vi "Hembras.vi"() -> ()   [LabVIEW 2013]
doc: "This example performs a serial port write and a serial port read. The parameters set for the serial port must match the parameters of the connected instrument or device. The VISA Configure Serial Port VI sets the configuration parameters. The front panel displays the controls used to configure the basic parameters, such as baud rate, data bits, and parity. The VI passes the VISA resource name to other VIs that perform operations on that VISA resource. The VISA Write function sends a command to the serial device and the VISA Read function returns data based on the command. The VISA Close function then closes the reference to the serial device. It is important to close the reference; otherwise, further communication through that port might not be possible."
uses:
  <vilib>/Platform/TimedLoop/XDataNode/timing_clust.ctl
  <vilib>/Platform/TimedLoop/XDataNode/nitl_modes.ctl
  <vilib>/Platform/TimedLoop/XDataNode/wakeup.ctl
  <vilib>/Instr/_visa.llb/VISA Configure Serial Port (Instr).vi
  <vilib>/Utility/file.llb/Read From Spreadsheet File (I64).vi
  <vilib>/platform/TimedLoop/XDataNode/XDataNode.xnode
  <vilib>/Platform/TimedLoop/XDataNode/XDNodeRunTimeDep.lvlib
panel:
  in  "Puerto":refnum<visa-resource-name>
  out "Entradas":u8[][](array[numeric])
  in  "Abrir arnés":bool
  out "Test":bool
  out "Bien?":bool[][](array[boolean])
  out "Entradas Testeadas":u8[][](array[numeric])
  out "Salidas":u8[](array[numeric])
  out "OK?":bool
  in  "stop":bool
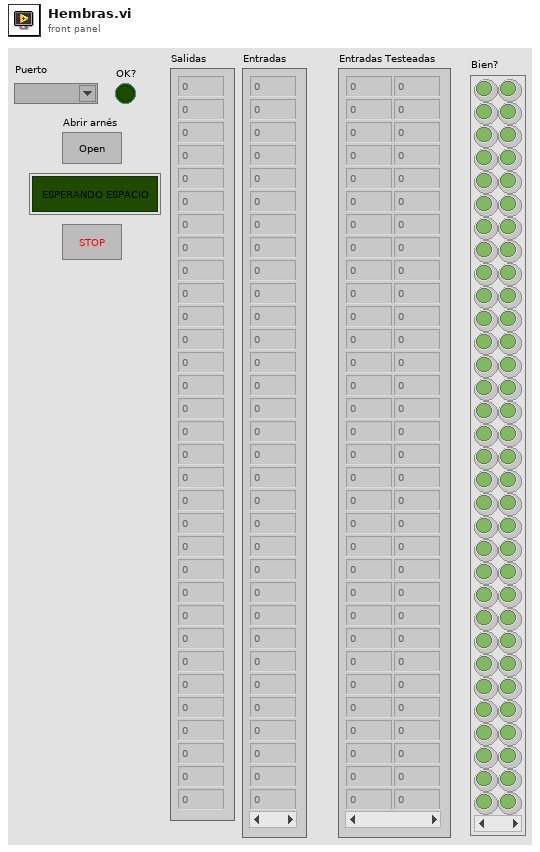
[diagram p1: front panel]
types:
  T1 = typedef "XDNodeRunTimeDep.lvlib/timing_clust.ctl" = cluster{"Expected End [f-1]":u64, "Actual End [f-1]":u64, "Finished Late? [f-1]":bool, "Expected End [i-1]":u64, "Actual End [i-1]":u64, "Finished Late? [i-1]":bool, "Expected Start [i]":u64, "Actual Start [i]":u64, "Expected Start [f]":u64, "Actual Start [f]":u64, "Source Name":string, "Structure Name":string, "Period":i64, "Deadline":i64, "Offset":i64, "Start":i64, "Priority":i32, "Timeout":i32, "Mode":T2, "Wakeup Reason":T3, "Error":errorcluster, "Source Type":string, "Secondary Source Type":string, "Global End Time":u64, "Global Start Time":u64, "Frame Duration":u64, "Iteration Duration":u64, "Assigned CPU":i32, "I/O Scan Engine Mode":u32}
  T2 = typedef "XDNodeRunTimeDep.lvlib/nitl_modes.ctl" = enum32{"No Change", "Process missed periods, maintain original phase", "Discard missed periods, maintain original phase", "Process missed periods, ignore original phase", "Discard missed periods, ignore original phase"}
  T3 = typedef "XDNodeRunTimeDep.lvlib/wakeup.ctl" = enum32{"Normal", "Aborted", "Asynchronous wakeup", "Timing source error", "Timed loop error", "Timeout"}
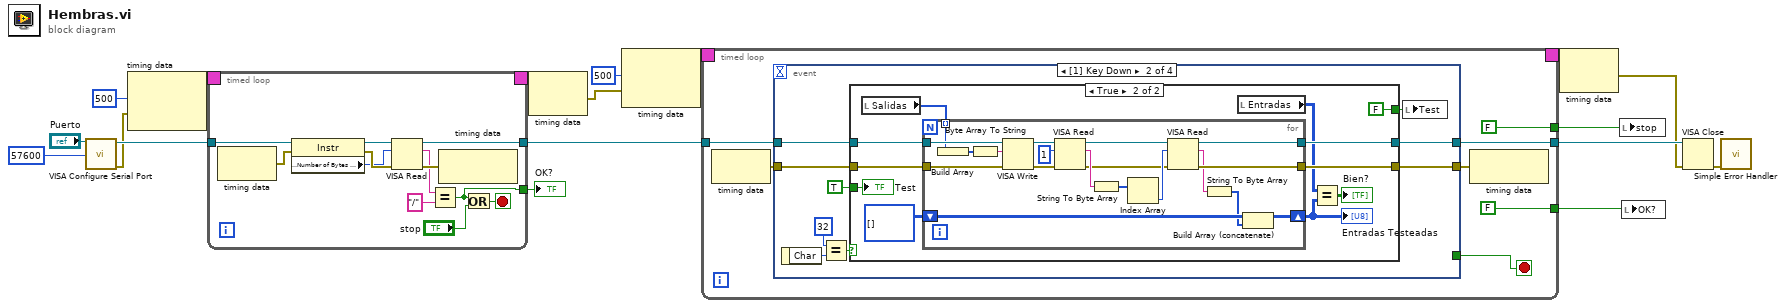
[diagram p0: block diagram]
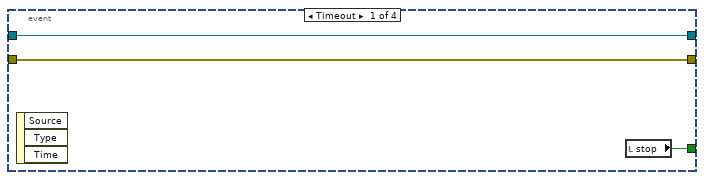
[diagram p2: hidden frame]
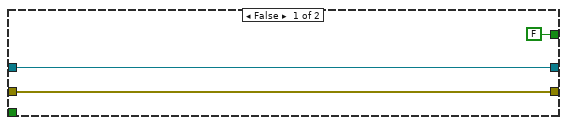
[diagram p3: hidden frame]
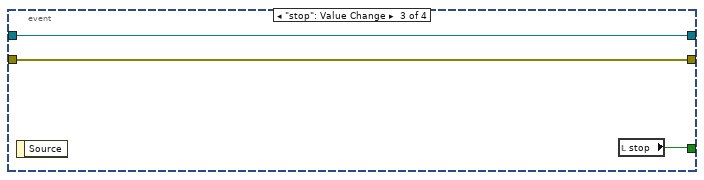
[diagram p4: hidden frame]
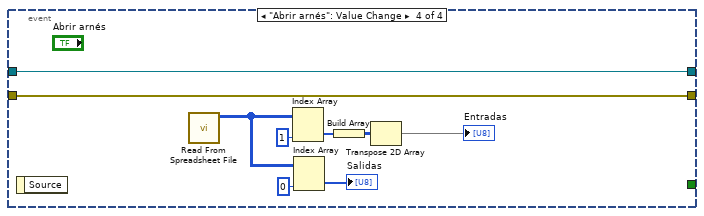
[diagram p5: hidden frame]
diagram:
  n1 = call-poly "VISA Configure Serial Port"("VISA resource name"="Puerto", "baud rate (9600)"=u32 57600) -> ("VISA resource name out"=w18:refnum<visa-resource-name>, "error out"=w15:errorcluster)  [unwired: 7 in, 5 out]
  n2 = node-c288(i64 500 ("Period"), w15) -> (w17:T1)
  n3 = timed-loop {
    timing: w17 -> [_]
    timing-out: [_] -> w16
    tunnel: [w30] -> w5
    tunnel: w18 -> [w29]
    tunnel: [w19] -> w8
    stop <- w20 stop-if-true
    n4 = node-c288() -> (w25:errorcluster)  [unwired: 1 in]
    n5 = property class="Instr"(reference=w29, error in=w25) -> (reference out=w28:refnum<visa-resource-name>, error out=w27:errorcluster, "Serial Settings:Number of Bytes at Serial Port"=w26:u32)
    n6 = VISA Read(VISA resource name=w28, byte count=w26, error in (no error)=w27) -> (VISA resource name out=w30:refnum<visa-resource-name>, read buffer=w23:string, error out=w24:errorcluster)  [unwired: 1 out]
    n7 = Equal?(x=w23, y="/") -> (x = y?=w19:bool)
    n8 = node-c288(w24) -> ()  [unwired: 1 out]
    n9 = Or(x=w19, y="stop") -> (x .or. y?=w20:bool)
  }
  "OK?" <- w8
  n10 = node-c288(w16) -> (w4:errorcluster)
  n11 = node-c288(i64 500 ("Period"), w4) -> (w11:T1)
  n12 = timed-loop {
    timing: w11 -> [_]
    timing-out: [_] -> w10
    tunnel: w5 -> [w42]
    tunnel: [FALSE ("stop")] -> w12
    tunnel: [w40] -> w3
    tunnel: [FALSE ("OK?")] -> w7
    stop <- w36 stop-if-true
    n13 = node-c288() -> (w39:errorcluster)  [unwired: 1 in]
    n14 = event shown="[1] Key Down" {
      selector: _ -> [_ _ _ _]
      dyn-events: _ -> [_ _ _ _]
      timeout: _ -> [_ _ _ _]
      tunnel: w42 -> [w44 w54 w89 w92]
      tunnel: [w44 w53 w89 w92] -> w40
      tunnel: w39 -> [w43 w52 w88 w91]
      tunnel: [w43 w51 w88 w91] -> w38
      tunnel: [w45 _ w90 _] -> w36
      event Timeout {
        n15 = event-data() -> ()  [unwired: 1 in, 3 out]
        n16 = local read "stop"() -> (w45:bool)
      }
      event Key Down {
        n17 = event-data() -> ("Char"=w49:i16)  [unwired: 1 in]
        n18 = Equal?(x=i16 32, y=w49) -> (x = y?=w50:bool)
        n19 = case shown="True" w50 {
          tunnel: w54 -> [w57 w68]
          tunnel: [w57 w65] -> w53
          tunnel: w52 -> [w56 w67]
          tunnel: [w56 w66] -> w51
          tunnel: TRUE -> [_ w61]
          tunnel: [FALSE FALSE] -> w46
          frame False {
          }
          frame True {
            n20 = local read "Salidas"() -> (w58:u8[])
            n21 = for {
              tunnel: w68 -> [w87]
              tunnel: w67 -> [w85]
              tunnel: [w77] -> w66
              tunnel: [w76] -> w65
              shift-right: [w74] -> w62
              shift-left: i32[][] [] -> [w73]
              tunnel: w58 -> [w69] mode=indexing
              n22 = Build Array(w69) -> (w71:u8[])
              n23 = Byte Array To String ("Byte Array \nTo String")(unsigned byte array=w71) -> (string=w70:string)
              n24 = VISA Write(VISA resource name=w87, write buffer=w70, error in (no error)=w85) -> (VISA resource name out=w84:refnum<visa-resource-name>, error out=w83:errorcluster)  [unwired: 1 out]
              n25 = VISA Read(VISA resource name=w84, byte count=u32 1, error in (no error)=w83) -> (VISA resource name out=w78:refnum<visa-resource-name>, read buffer=w86:string, error out=w79:errorcluster)  [unwired: 1 out]
              n26 = String To Byte Array(string=w86) -> (unsigned byte array=w81:u8[])
              n27 = Index Array(array=w81) -> (element=w80:u8)  [unwired: 1 in]
              n28 = VISA Read(VISA resource name=w78, byte count=w80, error in (no error)=w79) -> (VISA resource name out=w76:refnum<visa-resource-name>, read buffer=w75:string, error out=w77:errorcluster)  [unwired: 1 out]
              n29 = String To Byte Array(string=w75) -> (unsigned byte array=w72:u8[])
              n30 = Build Array (concatenate)(w73, w72) -> (w74:i32[][])
            }
            "Entradas Testeadas" <- w62
            n31 = local read "Entradas"() -> (w59:u8[][])
            n32 = Equal?(x=w59, y=w62) -> (x = y?=→"Bien?":bool[][])
            "Test" <- w61
          }
        }
        n33 = local write "Test"(w46) -> ()
      }
      event "stop": Value Change {
        n34 = event-data() -> ()  [unwired: 1 in, 1 out]
        n35 = local read "stop"() -> (w90:bool)
      }
      event "Abrir arnés": Value Change {
        n36 = event-data() -> ()  [unwired: 1 in, 1 out]
        n37 = call-poly <vilib>:"Read From Spreadsheet File.vi"() -> ("all rows"=w95:i64[][])  [unwired: 7 in, 4 out]
        n38 = Index Array(array=w95, index (col)=1 ("index (row)")) -> (element=w98:i64[])  [unwired: 1 in]
        n39 = Index Array(array=w95, index (col)=0 ("index (row)")) -> (element=→"Salidas":i64[])  [unwired: 1 in]
        n40 = Build Array(w98) -> (w97:i64[][])
        n41 = Transpose 2D Array(2D array=w97) -> (transposed array=→"Entradas":i64[][])
      }
    }
    n42 = node-c288(w38) -> ()  [unwired: 1 out]
  }
  n43 = node-c288(w10) -> (w2:errorcluster)
  n44 = local write "stop"(w12) -> ()
  n45 = local write "OK?"(w7) -> ()
  n46 = VISA Close(VISA resource name=w3, error in (no error)=w2) -> (error out=w13:errorcluster)
  n47 = call <vilib>:"Simple Error Handler.vi"("error in (no error)"=w13) -> ()  [unwired: 4 in, 5 out]
